vi "GetError-UiThread.vi"(8 "No Error":errorcluster) -> (0 "error out":errorcluster)   [LabVIEW 2026, in "SDL3.lvlib" / "Error.lvlib"]
doc: "<B>LV Implementation Note</B>\nAs stated by the function doc, error strings are thread specific, that's why where are two GetError vi. One for UI Thread calls, the other for any thread.\n\n<B>Summary</B>\nRetrieve a message about the last error that occurred on the current thread.\n\n<B>Remarks</B>\nIt is possible for multiple errors to occur before calling SDL_GetError(). Only the last error is returned.\n\nThe message is only applicable when an SDL function has signaled an error. You must check the return values of SDL function calls to determine when to appropriately call SDL_GetError(). You should not use the results of SDL_GetError() to decide if an error has occurred! Sometimes SDL will set an error string even when reporting success.\n\nSDL will not clear the error string for successful API calls. You must check return values for failure cases before you can assume the error string applies.\n\nError strings are set per-thread, so an error set in a different thread will not interfere with the current thread's operation.\n\nThe returned value is a thread-local string which will remain valid until the current thread's error string is changed. The caller should make a copy if the value is needed after the next SDL API call."
uses:
  Error.lvlib
  Lib/SDL3.dll
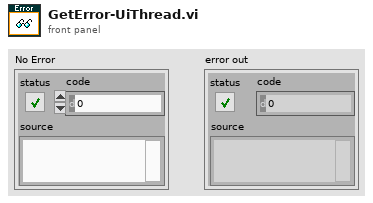
[diagram p1: front panel]
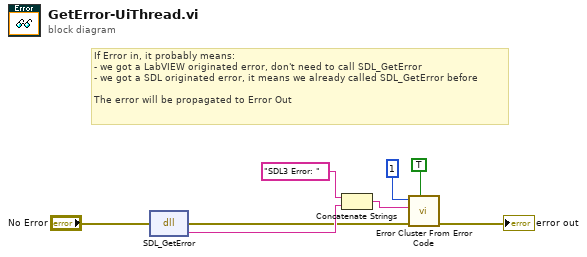
[diagram p0: block diagram]
diagram:
  # "If Error in, it probably means: \n- we got a LabVIEW originated error, don't need to call SDL_GetError\n- we got a SDL originated error, it means we already called SDL_GetError before\n\nThe error will be propagated to Error Out"
  n1 = dll-call lib="C:/Users/saukko/Dev/LV-SDL3/Sources/SDL3/Lib/SDL3.*" fn="SDL_GetError"(error in="No Error") -> (error out=w1:errorcluster, "return type"=w4:string)  [unwired: 2 in, 1 out]
  n2 = Concatenate Strings("SDL3 Error: " ("string"), w4) -> (w6:string)
  n3 = call <vilib>:"Error Cluster From Error Code.vi"("show call chain? (False)"=TRUE, "error in (no error)"=w1, "error message (\"\")"=w6, "error code (0)"=1) -> ("error out"=→"error out":errorcluster)  [unwired: 5 in]
